vi "read.vi"(8 "error in (no error)":errorcluster, 11 "Instrument in":refnum<class "AnalogReadSim.lvclass">) -> (0 "error out":errorcluster, 2 "outputs":dbl[](array[numeric]), 3 "Instrument out":refnum<class "AnalogReadSim.lvclass">)   [LabVIEW 2017, in "AnalogReadSim.lvclass"]
doc: "Read data from the instrument"
uses:
  AnalogReadSim.lvclass
  support/my_global.vi
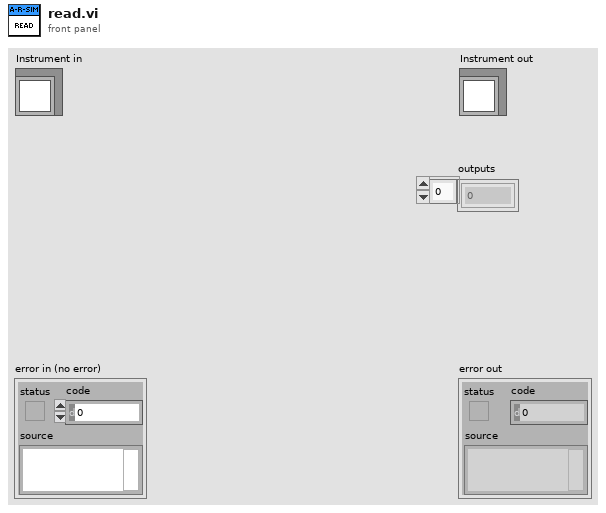
[diagram p1: front panel]
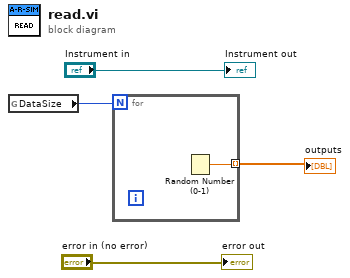
[diagram p0: block diagram]
diagram:
  n1 = global read "my_global.vi" "DataSize"() -> (w1:u32)
  n2 = for {
    N: w1 -> [_]
    tunnel: [w5] -> w2 mode=indexing
    n3 = Random Number (0-1)() -> (number: 0 to 1=w5:dbl)
  }
  "outputs" <- w2
  "error out" <- "error in (no error)"
  "Instrument out" <- "Instrument in"
